vi "FFT_averaging_debug.vi"(0 "dt":dbl, 1 "chirp end":dbl, 2 "frame":i32, 3 "current frequency":dbl, 8 "reset frame average":bool, 10 "all frames?":bool) -> (9 "BG waveform":waveform(dbl), 11 "Mol waveform":waveform(dbl), 12 "averages compl":i32, 13 "cor waveform":waveform(dbl), 14 "BG spectrum":T2, 16 "Mol spectrum":T2(graph), 18 "cor spectrum":T2(graph))   [LabVIEW 2011]
uses:
  global.vi
panel:
  in  "output cluster":T1
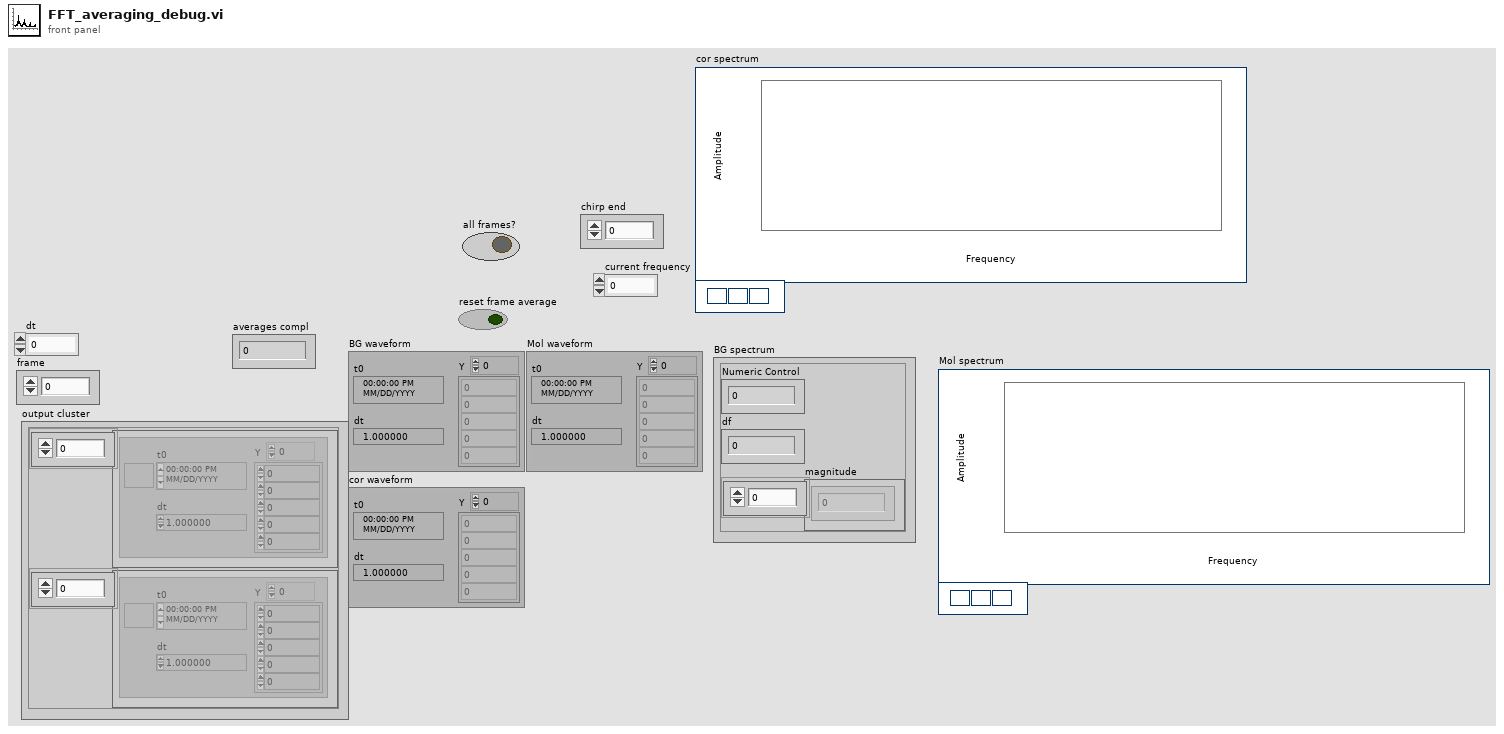
[diagram p1: front panel]
types:
  T1 = cluster{"Array":waveform(dbl)[], "Array":waveform(dbl)[]}
  T2 = cluster{"Numeric Control":dbl, "df":dbl, "magnitude":dbl[]}
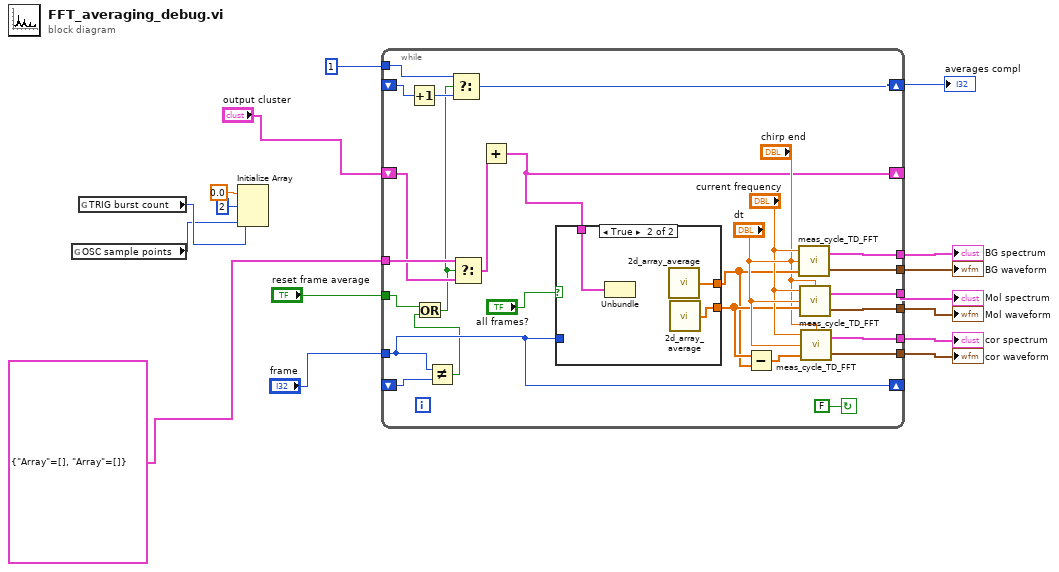
[diagram p0: block diagram]
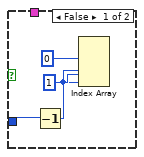
[diagram p2: hidden frame]
diagram:
  n1 = global read "global.vi" "OSC sample points"() -> (w13:i32)
  n2 = global read "global.vi" "TRIG burst count"() -> (w15:i32)
  n3 = Initialize Array(0.0 ("element"), 2 ("dimension size"), w15, w13) -> ()  [unwired: 1 out]
  n4 = while {
    shift-right: [w17] -> _
    shift-left: "output cluster" -> [w41]
    tunnel: T1 {"Array"=[], "Array"=[]} ("output cluster 2") -> [w42]
    tunnel: "reset frame average" -> [w20]
    shift-right: [w34] -> w11
    shift-left: _ -> [w39]
    tunnel: 1 -> [w37]
    tunnel: [w35] -> w10
    tunnel: [w36] -> w9
    tunnel: [w27] -> w7
    tunnel: [w26] -> w6
    tunnel: [w25] -> w5
    tunnel: [w24] -> w4
    tunnel: "frame" -> [w21]
    shift-right: [w21] -> _
    shift-left: _ -> [w22]
    stop <- FALSE continue-if-true
    n5 = Increment(x=w39) -> (x+1=w38:i32)
    n6 = Not Equal?(x=w21, y=w22) -> (x != y?=w18:bool)
    n7 = Or(x=w20, y=w18) -> (x .or. y?=w19:bool)
    n8 = Select(t=w37, s=w19, f=w38) -> (s? t:f=w34:i32)
    n9 = Select(t=w42, s=w19, f=w41) -> (s? t:f=w40:T1)
    n10 = Add(y=w40) -> (x+y=w17:T1)  [unwired: 1 in]
    n11 = case shown="True" "all frames?" {
      tunnel: [_ w49] -> w30
      tunnel: w21 -> [w44 _]
      tunnel: [_ w50] -> w29
      tunnel: w17 -> [_ w48]
      frame False {
        n12 = Decrement(x=w44) -> (x-1=w45:i32)
        n13 = Index Array(index (row) #1=0 ("disabled index (page)"), index (col) #1=w45, index (row) #2=1 ("disabled index (page)"), index (col) #2=w45) -> ()  [unwired: 1 in, 2 out]
      }
      frame True {
        n14 = Unbundle(w48) -> ()  [unwired: 2 out]
        n15 = call "2d_array_average.vi"() -> ("array average"=w50:dbl[])  [unwired: 5 in]
        n16 = call "2d_array_average.vi"() -> ("array average"=w49:dbl[])  [unwired: 5 in]
      }
    }
    n17 = Subtract(x=w30, y=w29) -> (x-y=w28:dbl[])
    n18 = call "meas_cycle_TD_FFT.vi"("chirp end"="chirp end", "time domain array"=w29, "dt"="dt", "current frequency"="current frequency") -> ("output time domain signal"=w26:waveform(dbl), "output spectrum"=w35:T2)
    n19 = call "meas_cycle_TD_FFT.vi"("chirp end"="chirp end", "time domain array"=w30, "dt"="dt", "current frequency"="current frequency") -> ("output time domain signal"=w25:waveform(dbl), "output spectrum"=w36:T2)
    n20 = call "meas_cycle_TD_FFT.vi"("chirp end"="chirp end", "time domain array"=w28, "dt"="dt", "current frequency"="current frequency") -> ("output time domain signal"=w24:waveform(dbl), "output spectrum"=w27:T2)
  }
  "averages compl" <- w11
  "Mol spectrum" <- w9
  "cor spectrum" <- w7
  "BG spectrum" <- w10
  "BG waveform" <- w6
  "Mol waveform" <- w5
  "cor waveform" <- w4
